vi "Set Sensitivity (V Mode).vi"(8 "error in (no error)":errorcluster, 10 "Sensitivity IMODE0":T1=enum."5 nV", 11 "VISA resource name":refnum<visa-resource-name>) -> (0 "error out":errorcluster, 3 "VISA resource name out":refnum<visa-resource-name>)   [LabVIEW 2016, in "SR7270 Drivers.lvlib"]
uses:
  SR7270 Drivers.lvlib
  Typedefs/SEN-IMODE0--enum.ctl
  Typedefs/IMODE--enum.ctl
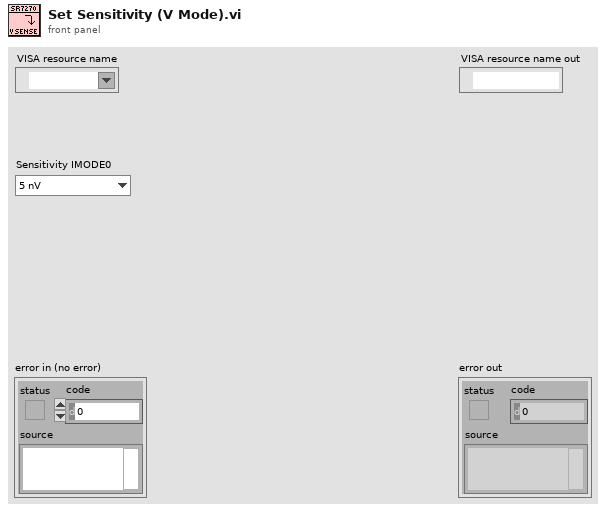
[diagram p1: front panel]
types:
  T1 = typedef "SR7270 Drivers.lvlib/SEN-IMODE0--enum.ctl" = enum16{"2 nV", "5 nV", "10 nV", "20 nV", "50 nV", "100 nV", "200 nV", "500 nV", "1 µV", "2 µV", "5 µV", "10 µV", "20 µV", "50 µV", "100 µV", "200 µV", "500 µV", "1 mV", "2 mV", "5 mV", "10 mV", "20 mV", "50 mV", "100 mV", "200 mV", "500 mV", "1 V"}
  T2 = typedef "SR7270 Drivers.lvlib/IMODE--enum.ctl" = enum16{"Current Mode Off", "High bandwidth current mode", "Low noise current mode"}
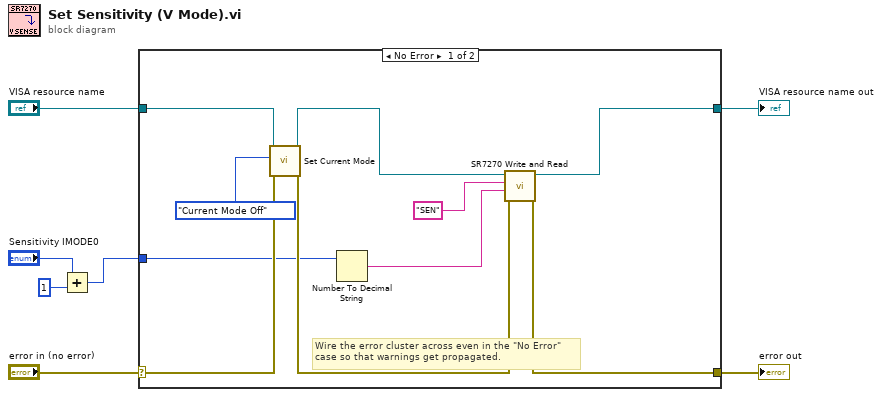
[diagram p0: block diagram]
diagram:
  n1 = Add(x="Sensitivity IMODE0", y=1) -> (x+y=w1:i32)
  n2 = case shown="No Error" "error in (no error)" {
    selector: "error in (no error)" -> [w15 w19]
    tunnel: [w13 w19] -> w7
    tunnel: [w8 w18] -> w6
    tunnel: "VISA resource name" -> [w10 w18]
    tunnel: w1 -> [w12 _]
    frame No Error {
      # "Wire the error cluster across even in the \"No Error\"\ncase so that warnings get propagated."
      n3 = call "Set Current Mode.vi"("error in (no error)"=w15, "Current Mode"=IMODE--enum."Current Mode Off", "VISA resource name"=w10) -> ("error out"=w14:errorcluster, "VISA resource name out"=w9:refnum<visa-resource-name>)  [unwired: 7 in]
      n4 = Number To Decimal String(number=w12) -> (decimal integer string=w11:string)  [unwired: 1 in]
      n5 = call "SR7270 Write and Read.vi"("error in (no error)"=w14, "Parameter(s)"=w11, "Command Name"="SEN", "VISA resource name"=w9) -> ("error out"=w13:errorcluster, "VISA resource name out"=w8:refnum<visa-resource-name>)  [unwired: 4 in, 2 out]
    }
    frame Error {
    }
  }
  "error out" <- w7
  "VISA resource name out" <- w6
